vi "Introspection Core.vi"(8 "error in (no error)":errorcluster, 11 "CS++GUIActor in":refnum<class "CS++GUIActor.lvclass">) -> (0 "error out":errorcluster, 2 "CS++Messages":refnum<class "Message.lvclass">[](array[class]), 3 "CS++GUIActor out":refnum<class "CS++GUIActor.lvclass">)   [LabVIEW 2014, in "CS++GUIActor.lvlib" / "CS++GUIActor.lvclass"]
doc: "This vi delivers a list with all messages this actor reacts to. \n\nNote that all inherited classes have to overwrite it."
uses:
  CS++GUIActor.lvclass
  CS++BaseActor/CS++BaseActor.lvclass
  <vilib>/ActorFramework/Message/Message.lvclass
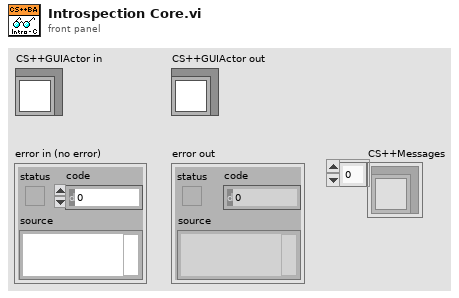
[diagram p1: front panel]
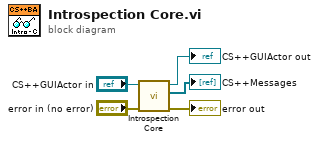
[diagram p0: block diagram]
diagram:
  n1 = call-parent "Introspection Core.vi"("error in (no error)"="error in (no error)", "CS++BaseActor in"="CS++GUIActor in") -> ("error out"=→"error out":errorcluster, "CS++Messages"=→"CS++Messages":refnum<class "Message.lvclass">[], "CS++BaseActor out"=→"CS++GUIActor out":refnum<class "CS++GUIActor.lvclass">)  [unwired: 7 in]
